vi "Write Tags.vi"(8 "error in (no error)":errorcluster, 11 "Agitator Module State Cluster":T1={"State"=enum."Idle", "Start Time"=timestamp(0 s since 1904-01-01), "Current Time"=timestamp(0 s since 1904-01-01), "Agitator Module Config"={"GUID"="", "Drop Coords"={"Horizontal"=0, "Vertical"=0}, "Process Name"="", "User name"="", "Queue Name"="", "Settings"={"Cycle Period"=500.0, "Agitator Type"="", "Setpoint (µm)"=0.0, "IKA EUROSTAR Settings"={"VISA resource name"="", "Simulated?"=FALSE}}, "Load Count"=0}, "Output Error"=FALSE, "Log Started"=FALSE, "First Iteration"=FALSE, "Data"={"Agitator rpm Value"=0.0}, "Agitator On?"=enum."Off"}) -> (0 "error out":errorcluster, 3 "Agitator Module State Cluster":T1={"State"=enum."Idle", "Start Time"=timestamp(0 s since 1904-01-01), "Current Time"=timestamp(0 s since 1904-01-01), "Agitator Module Config"={"GUID"="", "Drop Coords"={"Horizontal"=0, "Vertical"=0}, "Process Name"="", "User name"="", "Queue Name"="", "Settings"={"Cycle Period"=500.0, "Agitator Type"="", "Setpoint (µm)"=0.0, "IKA EUROSTAR Settings"={"VISA resource name"="", "Simulated?"=FALSE}}, "Load Count"=0}, "Output Error"=FALSE, "Log Started"=FALSE, "First Iteration"=FALSE, "Data"={"Agitator rpm Value"=0.0}, "Agitator On?"=enum."Off"})   [LabVIEW 2018, in "Agitator Module.lvlib" / "Agitator Module Engine.lvlib"]
uses:
  Agitator Module Engine.lvlib
  Feed Module/Controls/Agitator Module State Cluster.ctl
  Pump Module Folder/Measure Instrument/State Enum.ctl
  Feed Module/Controls/Agitator Module Config Cluster.ctl
  <vilib>/Utility/miscctls.llb/LVPoint32TypeDef.ctl
  Feed Module/Controls/Agitator Module Settings Cluster.ctl
  IKA EUROSTAR/IKA EUROSTAR Settings.ctl
  Shared Variables/Dynamic Shared Variables.lvlib
  Tag VIs/Tag FGV Operation Enum.ctl
  Agitator Module.lvlib
  Pump Module Folder/Measure Instrument/Pump Module Engine.lvlib
  IKA EUROSTAR/IKA EUROSTAR.lvlib
panel:
  # "Agitator Settings"
  # "Agitator Settings"
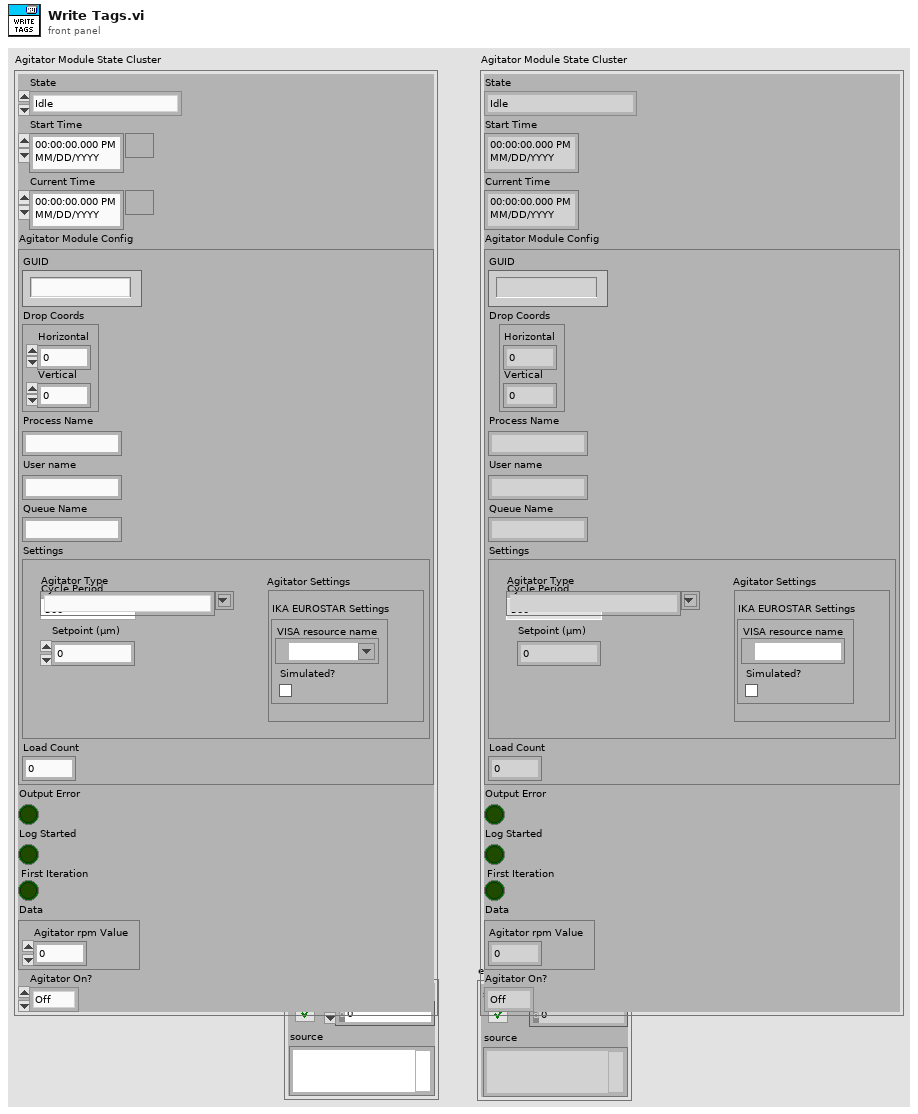
[diagram p1: front panel]
types:
  T1 = typedef "Agitator Module.lvlib/Agitator Module State Cluster.ctl" = cluster{"State":T2, "Start Time":timestamp, "Current Time":timestamp, "Agitator Module Config":T3, "Output Error":bool, "Log Started":bool, "First Iteration":bool, "Data":cluster{"Agitator rpm Value":dbl}, "Agitator On?":enum16{"Off", "On", "Not Initialized", "Over Cutoff"}}
  T2 = typedef "Pump Module.lvlib/Pump Module Engine.lvlib/State Enum.ctl" = enum16{"Measuring", "Idle", "Paused"}
  T3 = typedef "Agitator Module.lvlib/Agitator Module Config Cluster.ctl" = cluster{"GUID":string, "Drop Coords":T4, "Process Name":string, "User name":string, "Queue Name":string, "Settings":T5, "Load Count":i32}
  T4 = typedef "LVPoint32TypeDef.ctl" = cluster{"Horizontal":i32, "Vertical":i32}
  T5 = typedef "Agitator Module.lvlib/Agitator Module Settings Cluster.ctl" = cluster{"Cycle Period":dbl, "Agitator Type":string, "Setpoint (µm)":dbl, "IKA EUROSTAR Settings":T6}
  T6 = typedef "IKA EUROSTAR.lvlib/IKA EUROSTAR Settings.ctl" = cluster{"VISA resource name":refnum<visa-resource-name>, "Simulated?":bool}
  T7 = typedef "Tag FGV Operation Enum.ctl" = enum16{"Init", "Set Notification Queue", "Create Tag", "Commit", "Write Tag (Numeric)", "Write Tag (Boolean)", "Read All Tags", "Read One Tag", "Delete Tag Category", "Set Alarm Parameters (Numeric)", "Set Alarm Parameters (Boolean)", "Enable All Alarms", "Disable All Alarms", "Delete All Tags", "Read Alarms", "Ack Alarm", "Read Alarm Parameters (Numeric)", "Read Alarm Parameters (Boolean)"}
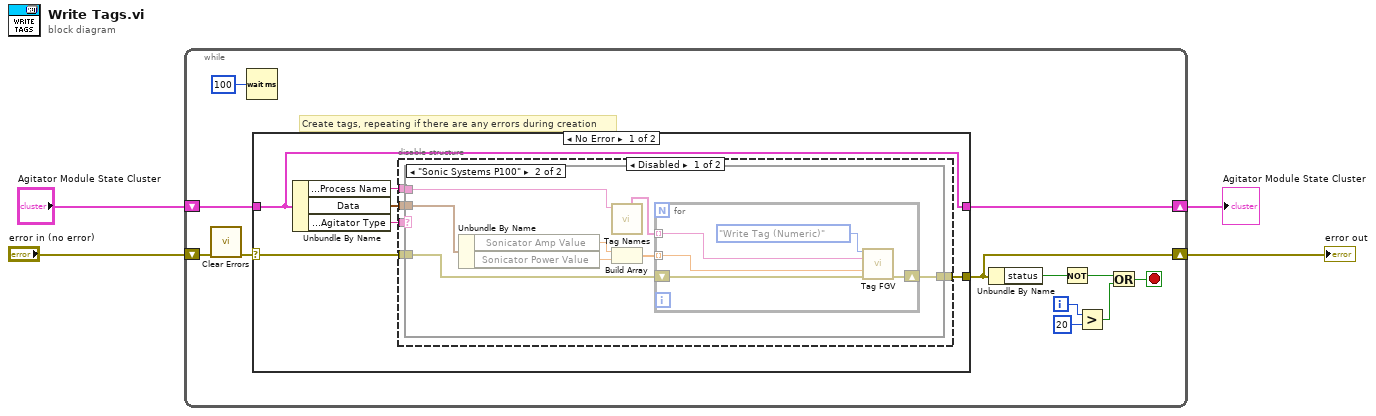
[diagram p0: block diagram]
diagram:
  n1 = while {
    shift-right: [w9] -> w3
    shift-left: "error in (no error)" -> [w14]
    shift-right: [w15] -> w1
    shift-left: "Agitator Module State Cluster" -> [w16]
    i -> [w7]
    stop <- w10 stop-if-true
    # "Create tags, repeating if there are any errors during creation"
    n2 = call <vilib>:"Clear Errors.vi"("error in (no error)"=w14) -> ("error out"=w13:errorcluster)  [unwired: 5 in, 1 out]
    n3 = Wait (ms)(milliseconds to wait=u32 100) -> ()  [unwired: 1 out]
    n4 = case shown="No Error" w13 {
      selector: w13 -> [w20 w43]
      tunnel: [w22 w43] -> w9
      tunnel: w16 -> [w21 w42]
      tunnel: [w21 w42] -> w15
      frame No Error {
        n5 = Unbundle By Name(w21) -> ("Agitator Module Config.Process Name"=w19:string, "Data"=w18:cluster{"Agitator rpm Value":dbl}, "Agitator Module Config.Settings.Agitator Type"=w17:string)
        n6 = disable-structure shown="Disabled" {
          disable-tunnel: [w27 _] -> w22
          disable-tunnel: w20 -> [w26 _]
          disable-tunnel: w19 -> [w25 _]
          disable-tunnel: w18 -> [w24 _]
          disable-tunnel: w17 -> [w23 _]
          frame Disabled {
            n7 = case shown="\"Sonic Systems P100\"" w23 {
              tunnel: [w28 w36] -> w27
              tunnel: w26 -> [w28 w35]
              tunnel: w25 -> [_ w34]
              tunnel: w24 -> [_ w32]
              frame Default {
              }
              frame "Sonic Systems P100" {
                n8 = Unbundle By Name(w32) -> ("Sonicator Amp Value"=w31:dbl, "Sonicator Power Value"=w30:dbl)
                n9 = call "Tag Names.vi"("Process Name"=w34) -> ("All  Numeric Tags"=w33:string[])  [unwired: 8 in, 2 out]
                n10 = Build Array(w31, w30) -> (w29:dbl[])
                n11 = for {
                  shift-right: [w41] -> w36
                  shift-left: w35 -> [w40]
                  tunnel: w33 -> [w37] mode=indexing
                  tunnel: w29 -> [w38] mode=indexing
                  n12 = call "Tag FGV.vi"("Operation"=Tag_FGV_Operation_Enum."Write Tag (Numeric)", "Tag Name"=w37, "Data"=w38, "error in (no error)"=w40) -> ("error out"=w41:errorcluster)  [unwired: 4 in, 7 out]
                }
              }
            }
          }
          frame Enabled {
          }
        }
      }
      frame Error {
      }
    }
    n13 = Unbundle By Name(w9) -> ("status"=w11:bool)
    n14 = Not(x=w11) -> (.not. x?=w12:bool)
    n15 = Greater?(x=w7, y=20) -> (0:w5:bool)
    n16 = Or(x=w12, y=w5) -> (x .or. y?=w10:bool)
  }
  "error out" <- w3
  "Agitator Module State Cluster" <- w1
